vi "Handle Framework Commands.vi"(8 "error in (no error)":errorcluster, 11 "Data Server Thread in":refnum<class "Data Server Thread.lvclass">) -> (0 "error out":errorcluster, 3 "Data Server Thread out":refnum<class "Data Server Thread.lvclass">)   [LabVIEW 2021, in "DSF Core.lvlib" / "Data Server Thread.lvclass"]
uses:
  Data Server Thread.lvclass
  C:/dev/git/custom-devices/niveristand-data-sharing-framework-custom-device/Source/Core/Classes/Thread/Thread.lvclass
  Data Server Thread.lvclass/Data Server Thread.ctl
  <vilib>/NI/Memory Manager/Classes/Pointer/Pointer.lvclass/Pointer.ctl
  Buffers/Buffers.lvclass/Buffers.ctl
  Buffer/Buffer.lvclass/Buffer.ctl
  Transfer/Transfer.lvclass/Transfer.ctl
  Thread.lvclass/Thread.ctl
  Interface/Errors.ctl
  <vilib>/NI/Memory Manager/Classes/Pointer/Encapsulate.vi
  Transfer/Align Buffers.vi
  Buffers/Align Inline Buffer.vi
  <vilib>/NI/Memory Manager/Classes/Pointer/Write.vi
  <vilib>/NI/Memory Manager/Classes/Pointer/Write Bool.vi
  <vilib>/NI/Memory Manager/Classes/Pointer/Set Size.vi
  <vilib>/NI/Memory Manager/Classes/Pointer/Set Address.vi
  <vilib>/NI/Memory Manager/Classes/Pointer/Check Null Pointer.vi
  <vilib>/NI/Memory Manager/Classes/Pointer/Set Internal.vi
  Buffers/Align Buffers.vi
  Buffer/Align to Base Buffer.vi
  <vilib>/NI/Memory Manager/Classes/Pointer/Write (No Check).vi
  <vilib>/NI/Memory Manager/Classes/Pointer/Write (No Check) Bool.vi
  <vilib>/NI/Memory Manager/Classes/Pointer/Check Move.vi
  <vilib>/NI/Memory Manager/Classes/Pointer/Errors.vi
  <vilib>/NI/Memory Manager/Classes/Pointer/Null Pointer.vi
  <vilib>/NI/Memory Manager/Classes/Pointer/Is Null.vi
  <vilib>/NI/Memory Manager/Classes/Pointer/Get Address.vi
  <vilib>/NI/Memory Manager/Classes/Pointer/Get Size.vi
  <vilib>/NI/Memory Manager/Classes/Pointer/Check Count.vi
  <vilib>/NI/Memory Manager/Classes/Pointer/Check Bounds (Power of 2).vi
  <vilib>/NI/Memory Manager/Classes/Pointer/Create Error.vi
  <vilib>/NI/Memory Manager/Classes/Pointer/Out of Bounds.vi
  <vilib>/NI/Memory Manager/Classes/Pointer/Check Bounds.vi
  <vilib>/NI/Memory Manager/VIs/New Error Cluster.vi
  <vilib>/NI/Memory Manager/VIs/New Error Cluster (512B).vi
  <vilib>/NI/Memory Manager/VIs/Set Error Status.vi
  <vilib>/NI/Memory Manager/VIs/Set Error Code.vi
  <vilib>/NI/Memory Manager/VIs/Set Error Source.vi
  <vilib>/NI/Memory Manager/Constants/Constants.vi
  <vilib>/NI/Memory Manager/Constants/Library Name.vi
  <vilib>/NI/Memory Manager/Classes/Pointer/Pointer Error Info.vi
  <vilib>/NI/Memory Manager/VIs/Write String to Source.vi
  <vilib>/NI/Memory Manager/Constants/Pointer Class Name.vi
  <vilib>/NI/Memory Manager/Classes/Pointer/Write Pointer Size to Error.vi
  <vilib>/NI/Memory Manager/VIs/Write Numeric to Source.vi
  <vilib>/NI/Memory Manager/VIs/Write Numeric Scalar to Source (Base10 U64).vi
  <vilib>/NI/Memory Manager/Classes/Pointer/Check Bounds (Pointer).vi
  <vilib>/NI/Memory Manager/Classes/Pointer/Check Bounds (Buffer).vi
  <vilib>/NI/Memory Manager/Classes/Pointer/Buffer Underflow.vi
  Buffer/Buffer.lvclass
  C:/Program Files/National Instruments/LabVIEW 2021/vi.lib/NI/Memory Manager/Classes/Pointer/Pointer.lvclass
  Interface/Plugin/Plugin Interface.lvclass
  C:/dev/git/custom-devices/niveristand-data-sharing-framework-custom-device/Source/Core/Classes/Interface/Interface.lvclass
  Interface/Interface.lvclass
  Thread.lvclass
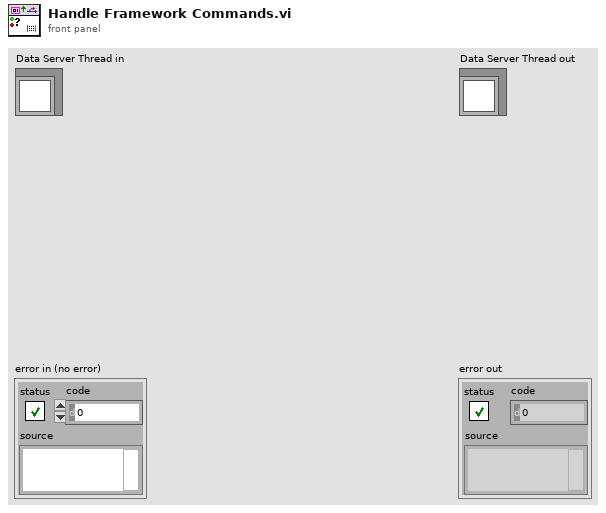
[diagram p1: front panel]
types:
  T1 = typedef "DSF Core.lvlib/Plugin Interface.lvclass/Command Data.ctl" = cluster{"Command":T2, "Parameters":T3}
  T2 = typedef "DSF Core.lvlib/Plugin Interface.lvclass/Command.ctl" = enum8{"Idle", "Start", "Set Inline Buffer", "Rx", "Tx", "Shutdown", "Error"}
  T3 = typedef "DSF Core.lvlib/Plugin Interface.lvclass/Command Parameters.ctl" = cluster{"arg1":u64, "arg2":u64}
  T4 = typedef "DSF Core.lvlib/Interface.lvclass/Errors.ctl" = enum16{"Command Timeout", "Response Timeout", "Error Timeout", "Invalid Response", "Invalid Response Parameters"}
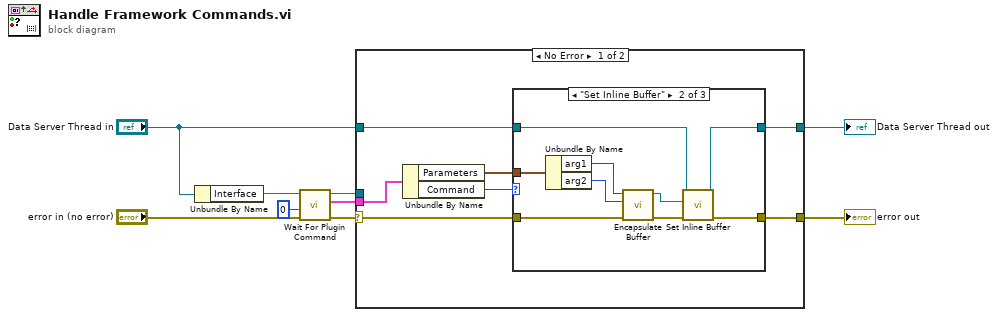
[diagram p0: block diagram]
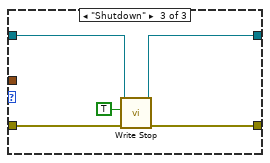
[diagram p3: hidden frame]
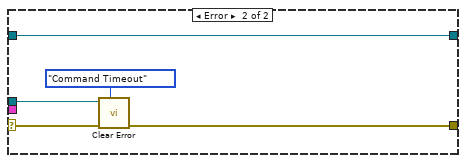
[diagram p4: hidden frame]
diagram:
  n1 = Unbundle By Name("Data Server Thread in") -> ("Interface"=w8:refnum<class "Plugin Interface.lvclass">)
  n2 = call "Wait For Plugin Command.vi"("error in (no error)"="error in (no error)", "timeout in ms (0)"=0, "Plugin Interface in"=w8) -> ("error out"=w4:errorcluster, "command"=w3:T1, "Plugin Interface out"=w5:refnum<class "Plugin Interface.lvclass">)  [unwired: 5 in, 1 out]
  n3 = case shown="No Error" w4 {
    selector: w4 -> [w14 w34]
    tunnel: [w13 w37] -> w6
    tunnel: w5 -> [_ w36]
    tunnel: w3 -> [w16 _]
    tunnel: "Data Server Thread in" -> [w11 w33]
    tunnel: [w10 w33] -> w1
    frame No Error {
      n4 = Unbundle By Name(w16) -> ("Parameters"=w12:T3, "Command"=w15:T2)
      n5 = case shown="\"Set Inline Buffer\"" w15 {
        tunnel: w14 -> [w18 w25 w29]
        tunnel: [w18 w19 w28] -> w13
        tunnel: w12 -> [_ w27 _]
        tunnel: w11 -> [w17 w23 w31]
        tunnel: [w17 w22 w30] -> w10
        frame "Idle", Default {
        }
        frame "Set Inline Buffer" {
          n6 = Unbundle By Name(w27) -> ("arg1"=w24:u64, "arg2"=w26:u64)
          n7 = call "Encapsulate Buffer.vi"("error in (no error)"=w25, "buffer size"=w26, "buffer address"=w24) -> ("error out"=w20:errorcluster, "Buffer"=w21:refnum<class "Buffer.lvclass">)  [unwired: 7 in]
          n8 = call "Set Inline Buffer.vi"("error in (no error)"=w20, "base Inline Buffer"=w21, "Data Server Thread in"=w23) -> ("error out"=w19:errorcluster, "Data Server Thread out"=w22:refnum<class "Data Server Thread.lvclass">)  [unwired: 7 in]
        }
        frame "Shutdown" {
          n9 = call "Write Stop.vi"("error in (no error)"=w29, "stop"=TRUE, "Thread in"=w31) -> ("error out"=w28:errorcluster, "Thread out"=w30:refnum<class "Data Server Thread.lvclass">)  [unwired: 7 in]
        }
      }
    }
    frame Error {
      n10 = call "Clear Error.vi"("error to clear"=Errors."Command Timeout", "error in (no error)"=w34, "Interface in"=w36) -> ("error out"=w37:errorcluster)  [unwired: 6 in, 2 out]
    }
  }
  "error out" <- w6
  "Data Server Thread out" <- w1
